vi "ones_2d.vi"(2 "m":i32=1, 3 "n":i32=1) -> (7 "ones":dbl[][](array[numeric]))   [LabVIEW 2017, in "NI_Gmath.lvlib"]
uses:
  NI_Gmath.lvlib
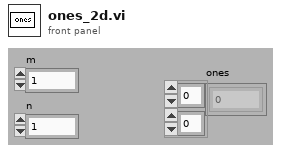
[diagram p1: front panel]
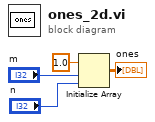
[diagram p0: block diagram]
diagram:
  n1 = Initialize Array(1.0 ("element"), "m", "n") -> (→"ones":dbl[][])
